vi "Run Tests.vi"(8 "error in":errorcluster, 11 "Report Path in":path) -> (0 "error out":errorcluster, 3 "Report Path Out":path)   [LabVIEW 2024, in "serenial.io-ase.test.lvlib"]
uses:
  serenial.io-ase.test.lvlib
  <vilib>/addons/_JKI Toolkits/Caraya/classes/Test Suite/Test Suite.lvclass
  <vilib>/addons/_JKI Toolkits/Caraya/classes/Test Suite/Define Test Suite (Default).vi
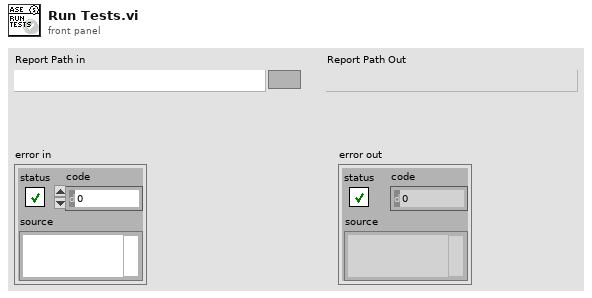
[diagram p1: front panel]
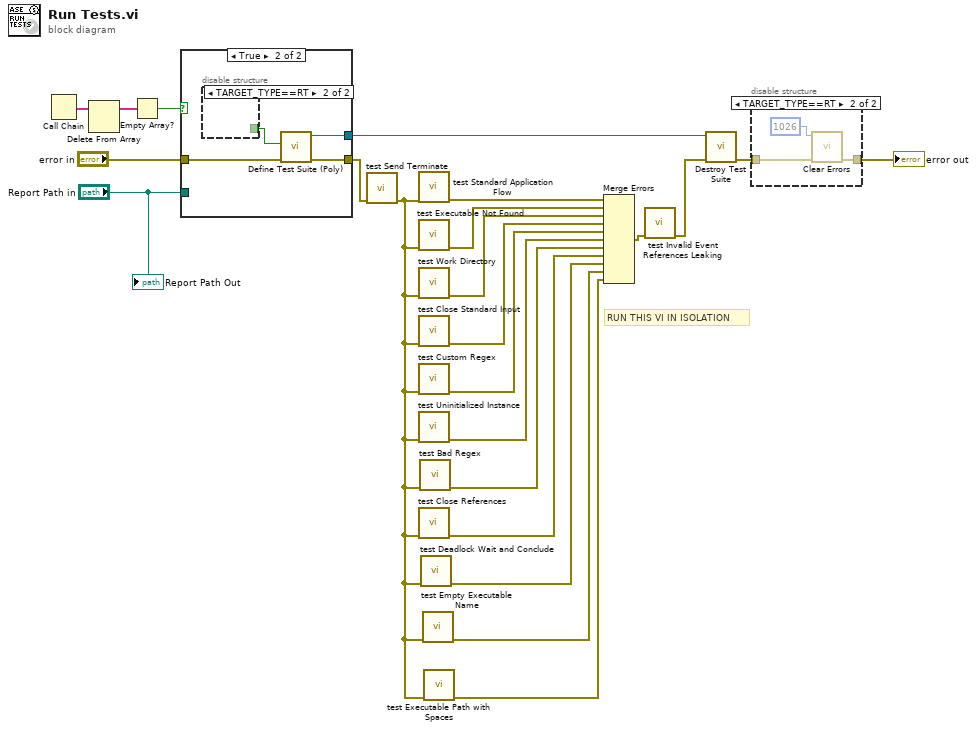
[diagram p0: block diagram]
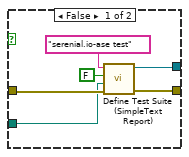
[diagram p3: hidden frame]
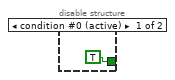
[diagram p4: hidden frame]
diagram:
  # "RUN THIS VI IN ISOLATION"
  n1 = Call Chain() -> (call chain=w15:string[])
  n2 = Delete From Array(array=w15) -> (array with subset deleted=w14:string[])  [unwired: 2 in, 1 out]
  n3 = Empty Array?(array=w14) -> (empty?=w13:bool)
  n4 = case shown="True" w13 {
    tunnel: "error in" -> [w27 w33]
    tunnel: [w29 w32] -> w16
    tunnel: [w28 w31] -> w9
    tunnel: "Report Path in" -> [w26 _]
    frame False {
      n5 = call <vilib>:"Define Test Suite (SimpleText Report).vi"("error in (no error)"=w27, "Report Path"=w26, "Interactive"=FALSE, "Label (VI Title)"="serenial.io-ase test") -> ("error out"=w28:errorcluster, "Test Suite"=w29:refnum<class "Test Suite.lvclass">)  [unwired: 5 in, 1 out]
    }
    frame True {
      n6 = disable-structure shown="TARGET_TYPE==RT" {
        disable-tunnel: [TRUE ("Interactive") _] -> w30
        frame condition #0 (active) {
        }
        frame condition #1 {
        }
      }
      n7 = call-poly <vilib>:"Define Test Suite (Poly).vi"("error in (no error)"=w33, "Interactive"=w30) -> ("error out"=w31:errorcluster, "Test Suite"=w32:refnum<class "Test Suite.lvclass">)  [unwired: 7 in, 1 out]
    }
  }
  n8 = call "test Send Terminate.vi"("error in"=w9) -> ("error out"=w4:errorcluster)  [unwired: 10 in]
  n9 = call "test Standard Application Flow.vi"("error in"=w4) -> ("error out"=w23:errorcluster)  [unwired: 10 in]
  n10 = call "test Executable Not Found.vi"("error in"=w4) -> ("error out"=w22:errorcluster)  [unwired: 10 in]
  n11 = call "test Work Directory.vi"("error in"=w4) -> ("error out"=w21:errorcluster)  [unwired: 10 in]
  n12 = call "test Close Standard Input.vi"("error in"=w4) -> ("error out"=w20:errorcluster)  [unwired: 10 in]
  n13 = call "test Custom Regex.vi"("error in"=w4) -> ("error out"=w19:errorcluster)  [unwired: 10 in]
  n14 = call "test Uninitialized Instance.vi"("error in"=w4) -> ("error out"=w18:errorcluster)  [unwired: 10 in]
  n15 = call "test Close References.vi"("error in"=w4) -> ("error out"=w10:errorcluster)  [unwired: 10 in]
  n16 = call "test Bad Regex.vi"("error in"=w4) -> ("error out"=w11:errorcluster)  [unwired: 10 in]
  n17 = call "test Deadlock Wait and Conclude.vi"("error in"=w4) -> ("error out"=w8:errorcluster)  [unwired: 10 in]
  n18 = call "test Empty Executable Name.vi"("error in"=w4) -> ("error out"=w5:errorcluster)  [unwired: 10 in]
  n19 = call "test Executable Path with Spaces.vi"("error in"=w4) -> ("error out"=w3:errorcluster)  [unwired: 10 in]
  n20 = Merge Errors(w23, w22, w21, w20, w19, w18, w11, w10, w8, w5, w3) -> (w7:errorcluster)
  n21 = call "test Invalid Event References Leaking.vi"("error in"=w7) -> ("error out"=w6:errorcluster)  [unwired: 10 in]
  n22 = call-dynamic "Destroy Test Suite.vi"("error in (no error)"=w6, "Test Suite in"=w16) -> ("error out"=w2:errorcluster)  [unwired: 8 in, 1 out]
  n23 = disable-structure shown="TARGET_TYPE==RT" {
    disable-tunnel: w2 -> [w35 w37]
    disable-tunnel: [w35 w38] -> w1
    frame condition #0 (active) {
    }
    frame condition #1 {
      n24 = call <vilib>:"Clear Errors.vi"("error in (no error)"=w37, "specific error code to clear (0: all)"=1026) -> ("error out"=w38:errorcluster)  [unwired: 4 in, 1 out]
    }
  }
  "error out" <- w1
  "Report Path Out" <- "Report Path in"
